vi "Start cameras.vi"(8 "Buffer size":i32, 11 "Camera 2?":bool) -> (0 "error out":errorcluster, 2 "error out 2":errorcluster, 3 "Refnum out":T2, 4 "Session Out":T2, 5 "Images Out 2":T1[](array[typedef]), 7 "Images Out":T1[](array[typedef]))   [LabVIEW 2018]
uses:
  <vilib>/userdefined/High Color/IMAQdx.ctl
  <vilib>/vision/Image Controls.llb/IMAQ Image.ctl
  <vilib>/vision/driver/NI_Vision_Acquisition_Software.lvlib
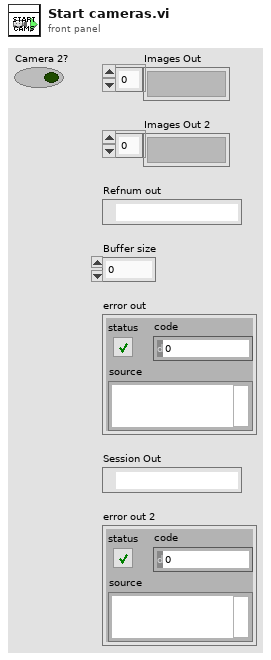
[diagram p1: front panel]
types:
  T1 = typedef "IMAQ Image.ctl" = refnum<image>
  T2 = typedef "IMAQdx.ctl" = refnum<k21>
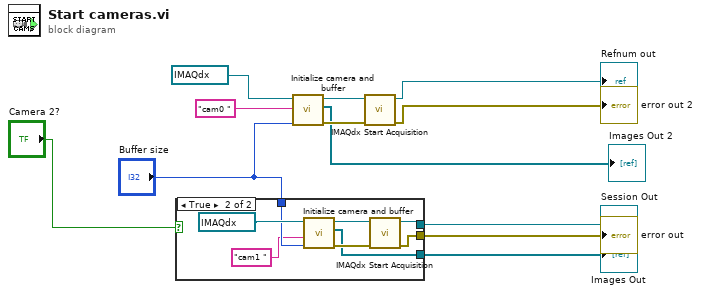
[diagram p0: block diagram]
diagram:
  n1 = case shown="True" "Camera 2?" {
    tunnel: "Buffer size" -> [_ w17]
    tunnel: [_ w16] -> w8
    tunnel: [_ w15] -> w9
    tunnel: [_ w14] -> w10
    frame False {
    }
    frame True {
      n2 = call "Initialize camera and buffer.vi"("Buffer size"=w17, "Image Name"="cam1 ", "Session In"=T2 "cam1") -> ("error out"=w19:errorcluster, "Images Out"=w16:T1[], "Session Out"=w20:T2)  [unwired: 6 in]
      n3 = call <vilib>:"IMAQdx Start Acquisition.vi"("error in"=w19, "Session In"=w20) -> ("error out"=w14:errorcluster, "Session Out"=w15:T2)  [unwired: 8 in]
    }
  }
  "error out" <- w10
  "Session Out" <- w9
  "Images Out" <- w8
  n4 = call "Initialize camera and buffer.vi"("Buffer size"="Buffer size", "Image Name"="cam0 ", "Session In"=T2 "cam0") -> ("error out"=w4:errorcluster, "Images Out"=→"Images Out 2":T1[], "Session Out"=w3:T2)  [unwired: 6 in]
  n5 = call <vilib>:"IMAQdx Start Acquisition.vi"("error in"=w4, "Session In"=w3) -> ("error out"=→"error out 2":errorcluster, "Session Out"=→"Refnum out":T2)  [unwired: 8 in]
